vi "logToFileTdms.vi"() -> ()   [LabVIEW 2017]
panel:
  out "Error Message":errorcluster
  in  "Stop Data Collection":bool
  out "Elapsed time <s>":dbl format="%#_13g"
  in  "PWM Command":dbl min=0.0 max=255.0 step=1.0
  out "Voltage Chart":waveform(dbl)(graph)
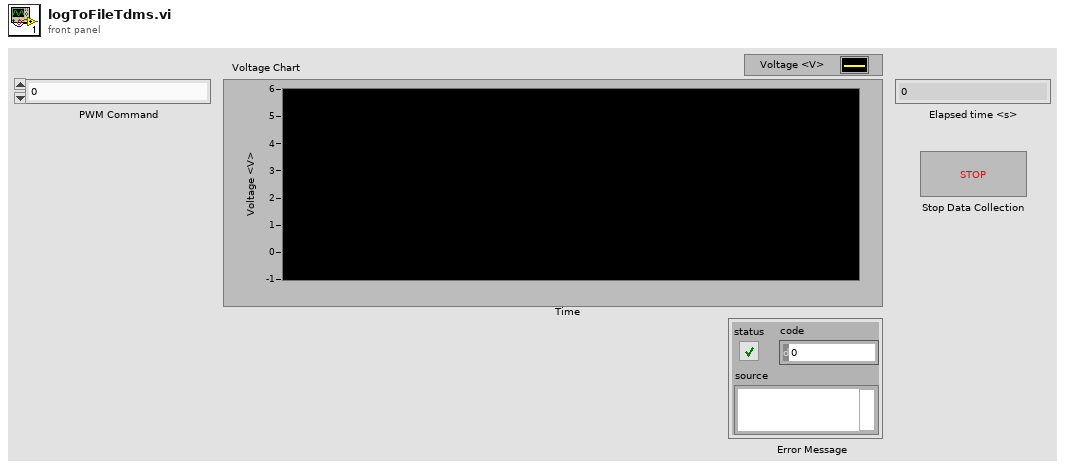
[diagram p1: front panel]
types:
  T1 = enum16{"open", "open or create", "create or replace", "create", "open (read-only)"}
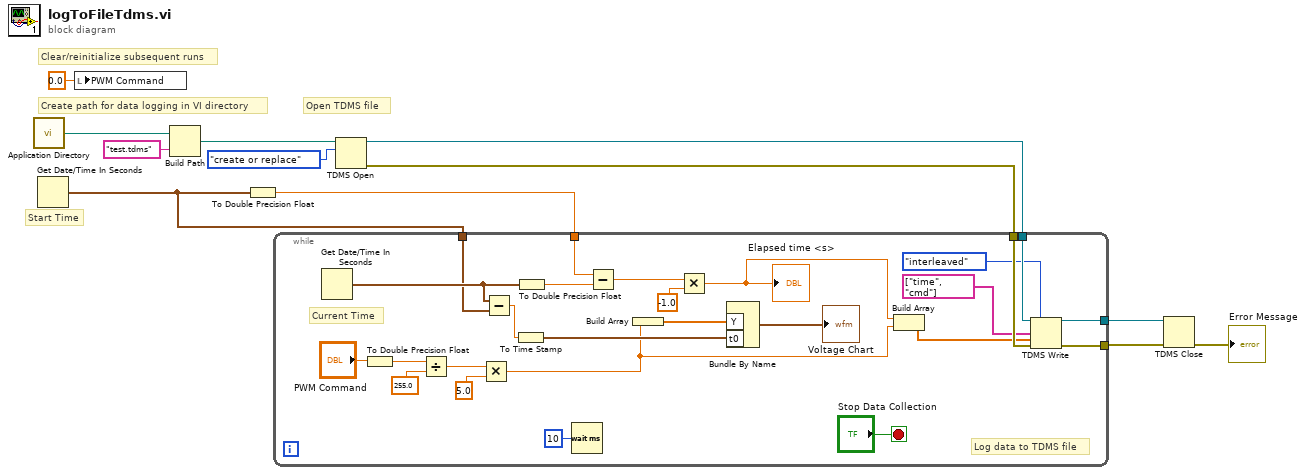
[diagram p0: block diagram]
diagram:
  # "Open TDMS file"
  # "Create path for data logging in VI directory"
  # "Clear/reinitialize subsequent runs"
  # "Start Time"
  n1 = call <vilib>:"Application Directory.vi"() -> ("Application Directory"=w3:path)
  n2 = Get Date/Time In Seconds() -> (seconds since 1Jan1904=w10:timestamp)
  n3 = local write "PWM Command"(0.0 ("PWM Command")) -> ()
  n4 = Build Path(base path=w3, name or relative path="test.tdms") -> (appended path=w2:path)
  n5 = To Double Precision Float(number=w10) -> (double precision float=w11:dbl)
  n6 = TDMS Open(10:T1."create or replace" ("operation (0:open)"), 11:w2) -> (0:w7:errorcluster, 3:w8:refnum<k34>)  [unwired: 5 in]
  n7 = while {
    tunnel: w11 -> [w33]
    tunnel: w10 -> [w25]
    tunnel: w8 -> [w20]
    tunnel: w7 -> [w19]
    tunnel: [w18] -> w6
    tunnel: [w17] -> w5
    stop <- "Stop Data Collection" stop-if-true
    # "Log data to TDMS file"
    # "Current Time"
    n8 = Get Date/Time In Seconds() -> (seconds since 1Jan1904=w26:timestamp)
    n9 = To Double Precision Float(number="PWM Command") -> (double precision float=w34:dbl)
    n10 = Divide(x=w34, y=255.0) -> (x/y=w37:dbl)
    n11 = Multiply(x=w37, y=5.0) -> (x*y=w21:dbl)
    n12 = Subtract(x=w26, y=w25) -> (x-y=w24:dbl)
    n13 = To Time Stamp(1:w24) -> (0:w23:timestamp)
    n14 = To Double Precision Float(number=w26) -> (double precision float=w29:dbl)
    n15 = Wait (ms)(milliseconds to wait=u32 10) -> ()  [unwired: 1 out]
    n16 = Subtract(x=w33, y=w29) -> (x-y=w32:dbl)
    n17 = Build Array(w21) -> (w28:dbl[])
    n18 = Multiply(x=w32, y=-1.0) -> (x*y=w22:dbl)
    "Elapsed time <s>" <- w22
    n19 = Bundle By Name("Y"=w28, "t0"=w23) -> (→"Voltage Chart":waveform(dbl))  [unwired: 1 in]
    n20 = Build Array(w22, w21) -> (w15:dbl[])
    n21 = TDMS Write(0:w20, 1:enum16{"decimated", "interleaved"}."interleaved" ("data layout (0:decimated)"), 7:string[] ["time", "cmd"] ("channel name(s) in (Untitled)"), 9:w15, 11:w19) -> (4:w18:refnum<k34>, 15:w17:errorcluster)  [unwired: 1 in, 2 out]
  }
  n22 = TDMS Close(8:w5, 11:w6) -> (0:→"Error Message":errorcluster)  [unwired: 1 out]
